vi "dfd_Get Filter Frequency Response from TF.vi"(4 "phase view":T1, 6 "fs [Hz]":dbl=1.0 format="%.2f", 7 "# freq bins (512)":i32=512, 8 "error in (no error)":errorcluster, 9 "magnitude":u16(ring) items=["Linear", "dB", "Zero phase"], 10 "den":dbl[](array[numeric])=[1.0] caption="denominator" format="%.2f", 11 "num":dbl[](array[numeric]) caption="numerator" format="%.2f") -> (0 "error out":errorcluster, 1 "df":dbl, 2 "phase":dbl[](array[numeric]) format="%.2f", 3 "magnitude":dbl[](array[numeric]) format="%.2f", 5 "X(w)":cdb[](array[numeric]))   [LabVIEW 2017, in "NI_DigFilterLicensed.lvlib"]
uses:
  <vilib>/addons/Digital Filter Design/NI_DigFilterLicensed.lvlib
  <vilib>/addons/Digital Filter Design/_Objects.llb/DFD Phase Setting.ctl
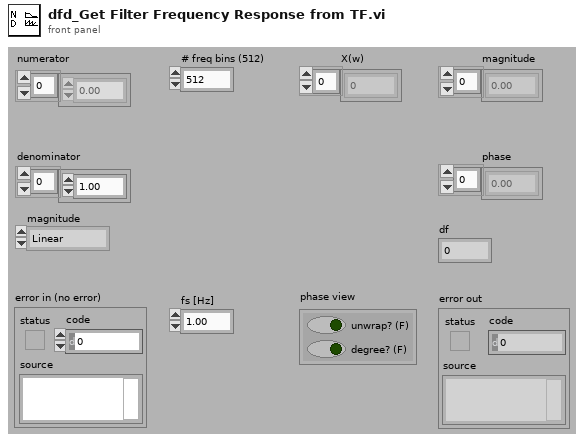
[diagram p1: front panel]
types:
  T1 = typedef "NI_DigFilterLicensed.lvlib/DFD Phase Setting.ctl" = cluster{"unwrap? (F)":bool, "degree? (F)":bool}
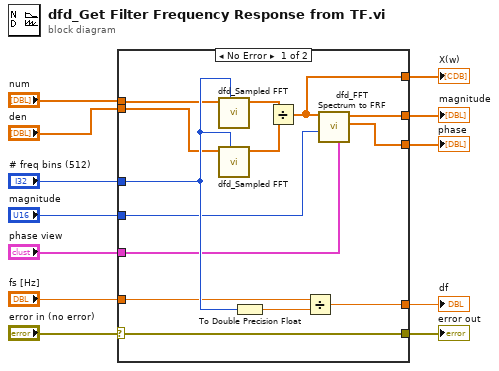
[diagram p0: block diagram]
diagram:
  n1 = case shown="No Error" "error in (no error)" {
    selector: "error in (no error)" -> [w14 w27]
    tunnel: [w19 _] -> w12
    tunnel: [w18 _] -> w11
    tunnel: "fs [Hz]" -> [w20 _]
    tunnel: "num" -> [w16 _]
    tunnel: "# freq bins (512)" -> [w25 _]
    tunnel: "phase view" -> [w22 _]
    tunnel: "magnitude" -> [w21 _]
    tunnel: "den" -> [w15 _]
    tunnel: [w14 w27] -> w3
    tunnel: [w17 _] -> w2
    tunnel: [w13 _] -> w1
    frame No Error {
      n2 = call <vilib>:"dfd_Sampled FFT.vi"("# freq bins (512)"=w25, "h[n]"=w16) -> ("FFT {X}"=w24:cdb[])  [unwired: 2 in, 7 out]
      n3 = call <vilib>:"dfd_Sampled FFT.vi"("# freq bins (512)"=w25, "h[n]"=w15) -> ("FFT {X}"=w23:cdb[])  [unwired: 1 in, 8 out]
      n4 = To Double Precision Float(number=w25) -> (double precision float=w26:dbl)
      n5 = Divide(x=w24, y=w23) -> (x/y=w13:cdb[])
      n6 = Divide(x=w20, y=w26) -> (x/y=w17:dbl)
      n7 = call <vilib>:"dfd_FFT Spectrum to FRF.vi"("phase view"=w22, "magnitude"=w21, "FFT {X}"=w13) -> ("phase"=w18:dbl[], "amplitude"=w19:dbl[])  [unwired: 3 in, 4 out]
    }
    frame Error {
    }
  }
  "magnitude" <- w12
  "phase" <- w11
  "error out" <- w3
  "df" <- w2
  "X(w)" <- w1
